vi "Update Channel Dependancy.vi"(8 "error in (no error)":errorcluster, 9 "NodeName":string, 10 "Data":variant, 11 "Item Ref in":T1 format="%.0x") -> (0 "error out":errorcluster, 3 "Item Ref out":T1 format="%.0x")   [LabVIEW 2015, in "Control Addon Shared.lvlib"]
uses:
  Control Addon Shared.lvlib
  <vilib>/NI Veristand/Custom Device API/Custom Device Item Ref.ctl
  NationalInstruments.VeriStand.SystemStorage
  <vilib>/NI Veristand/Custom Device API/Set Item Property (Dependent Node Pointer).vi
  <vilib>/NI VeriStand/Custom Device API/Custom Device API.lvlib
  <vilib>/NI Veristand/UI Controls/Single Node Browser/NI_VS UI Single Node Browser.lvlib
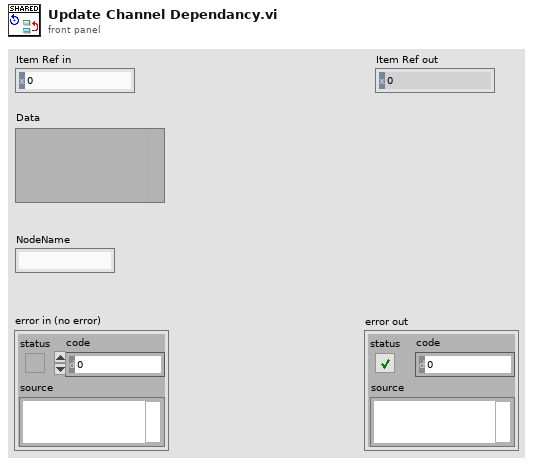
[diagram p1: front panel]
types:
  T1 = typedef "Custom Device API.lvlib/Custom Device Item Ref.ctl" = u64
  T2 = typedef "NI_VS UI Single Node Browser.lvlib/Node Ref.ctl" = refnum<k24>
  T3 = typedef "Custom Device API.lvlib/Custom Device Pointer.ctl" = refnum<k24>
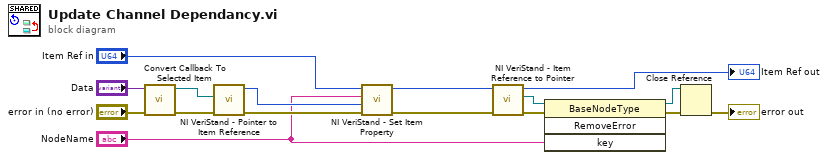
[diagram p0: block diagram]
diagram:
  n1 = call <vilib>:"Convert Callback To Selected Item.vi"("error in"="error in (no error)", "Data"="Data") -> ("error out"=w5:errorcluster, "Selected Item"=w10:T2)  [unwired: 8 in]
  n2 = call <vilib>:"NI VeriStand - Pointer to Item Reference.vi"("error in (no error)"=w5, "Node Pointer"=w10) -> ("error out"=w4:errorcluster, "Item Ref out"=w3:T1)  [unwired: 8 in]
  n3 = call-poly <vilib>:"NI VeriStand - Set Item Property.vi"("error in (no error)"=w4, "Dependent Node Ref"=w3, "Property Name"="NodeName", "Item Ref in"="Item Ref in") -> ("error out"=w6:errorcluster, "Item Ref out"=w7:T1)  [unwired: 5 in, 1 out]
  n4 = call <vilib>:"NI VeriStand - Item Reference to Pointer.vi"("error in (no error)"=w6, "Item Ref in"=w7) -> ("error out"=w15:errorcluster, "Node Pointer"=w16:T3, "Item Ref out"=→"Item Ref out":T1)  [unwired: 6 in, 1 out]
  n5 = invoke class="BaseNodeType" method="RemoveError"(reference=w16, error in=w15, "key"="NodeName") -> (reference out=w13:T3, error out=w14:errorcluster)  [unwired: 1 in, 2 out]
  n6 = Close Reference(reference=w13, error in (no error)=w14) -> (error out=→"error out":errorcluster)
